vi "SampleHTGyro.vi"   [LabVIEW 2016]
uses:
  <vilib>/NXT/HiTechnic/HiTechnic Controls/HiTechnic Port.ctl
  <vilib>/NXT/Block Support/NXT_InputPort.ctl
  <vilib>/NXT/Dual Mode Library/Display/drawText.vi
  <vilib>/NXT/Dual Mode Library/Waits/Wait_Num.vi
  <vilib>/NXT/Dual Mode Library/Waits/Wait_Num(msec).vi
  <vilib>/NXT/Dual Mode Library/Display/drawNumber.vi
types:
  T1 = typedef "HiTechnic Port.ctl" = cluster{"Port":T2, "MUX Port":u8}
  T2 = typedef "NXT_InputPort.ctl" = u32
  T3 = typedef "LVHSConnector.ctl" = refnum<class "BrickReference.lvclass">
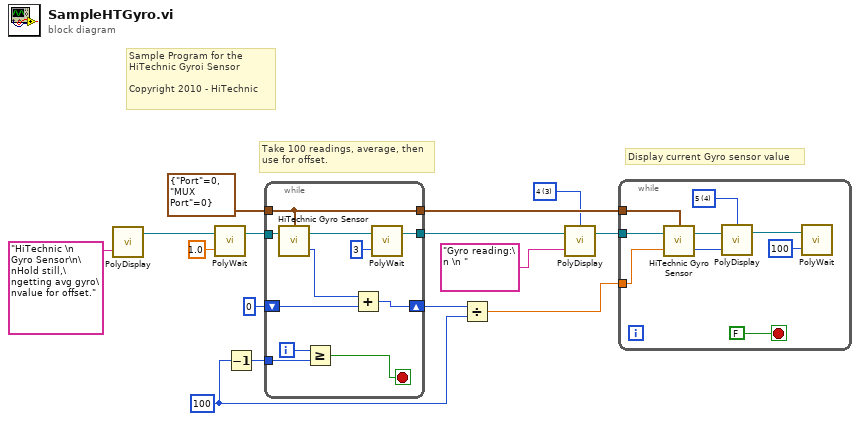
[diagram p0: block diagram]
diagram:
  w2 = i16 3 items=["1", "2", "3", "4", "5", "6", "7", "8"] ("Line")
  w12 = i16 100
  # "Display current Gyro sensor value"
  # "Take 100 readings, average, then\nuse for offset."
  # "Sample Program for the\nHiTechnic Gyroi Sensor\n\nCopyright 2010 - HiTechnic"
  n1 = call-poly <vilib>:"PolyDisplay.vi"("Text"="HiTechnic \n  Gyro Sensor\n\nHold still,\ngetting avg gyro\nvalue for offset.") -> ("NXT/EV3"=w6:T3)  [unwired: 3 in]
  n2 = call-poly <vilib>:"PolyWait.vi"("Time (1 sec)"=sgl 1.0 ("Time (sec)"), "NXT/EV3"=w6) -> ("NXT/EV3"=w7:T3)  [unwired: 2 in]
  n3 = Decrement(x=w12) -> (x-1=w14:i16)
  n4 = while {
    shift-right: [w24] -> w13
    shift-left: 0 -> [w25]
    tunnel: w14 -> [w22]
    tunnel: [w20] -> w3
    tunnel: T1 {"Port"=0, "MUX Port"=0} ("Port/MUX") -> [w17]
    tunnel: [w17] -> w9
    tunnel: w7 -> [w16]
    i -> [w23]
    stop <- w21 stop-if-true
    n5 = call <vilib>:"HiTechnic Gyro Sensor.vi"("NXT/EV3"=w16, "Port/MUX"=w17) -> ("Gyro Value"=w26:i16, "NXT/EV3"=w18:T3)  [unwired: 1 in]
    n6 = Greater Or Equal?(x=w23, y=w22) -> (x >= y?=w21:bool)
    n7 = Add(x=w26, y=w25) -> (x+y=w24:i32)
    n8 = call-poly <vilib>:"PolyWait.vi"("Time (100 msec)"=u32 3 ("Time (sec)"), "NXT/EV3"=w18) -> ("NXT/EV3"=w20:T3)  [unwired: 2 in]
  }
  n9 = Divide(x=w13, y=w12) -> (x/y=w11:dbl)
  n10 = call-poly <vilib>:"PolyDisplay.vi"("Text"="Gyro reading:\n \n ", "NXT/EV3"=w3, "Line"=w2) -> ("NXT/EV3"=w5:T3)  [unwired: 1 in]
  n11 = while {
    tunnel: w11 -> [w35]
    tunnel: w5 -> [w34]
    tunnel: w9 -> [w32]
    stop <- FALSE stop-if-true
    w30 = i16 4 items=["1", "2", "3", "4", "5", "6", "7", "8"] ("Line")
    n12 = call <vilib>:"HiTechnic Gyro Sensor.vi"("Offset"=w35, "NXT/EV3"=w34, "Port/MUX"=w32) -> ("Gyro Value"=w31:i16, "NXT/EV3"=w33:T3)
    n13 = call-poly <vilib>:"PolyDisplay.vi"("number"=w31, "NXT/EV3"=w33, "Line"=w30) -> ("NXT/EV3"=w27:T3)  [unwired: 1 in]
    n14 = call-poly <vilib>:"PolyWait.vi"("Time (100 msec)"=u32 100 ("Time (sec)"), "NXT/EV3"=w27) -> ()  [unwired: 2 in, 1 out]
  }
